vi "Design N IIR filters.vi"(4 "arrOptionalFilterSpecs":T3(array[cluster]) {"PB Gain" format="%0.2f"; "SB Gain" format="%0.2f"; "Lower SB" format="%0.2p"; "Upper SB" format="%0.2f"; "Lower PB" format="%0.2p"; "Upper PB" format="%0.2f"}, 6 "arrFilterSpecs":T2(array[cluster]) {"PB Ripple" format="%0.2f"; "Lower Fc" format="%0.2p"; "SB Attenuation" format="%0.2f"; "Upper Fc" format="%0.2p"}, 7 "redesign filters":bool[](array[boolean]), 8 "error in":errorcluster, 10 "filter structure option":T1=10 items=["IIR 2nd Order"=0, "IIR 4th Order"=1, "Auto Select"=10], 11 "arrdt":dbl[](array[numeric]) format="%0.2f") -> (0 "error out":errorcluster, 1 "arrIIRFilterCluster":T4(array[cluster]) {"Forward Coefficients" format="%0.2f"; "Reverse Coefficients" format="%0.2f"}, 3 "arrFilterInfo":T5(array[cluster]) {"phase H(w)"."df" format="%0.2f"; "phase H(w)"."f0" format="%0.2f"; "phase H(w)"."Phase H(w)" format="%0.2f"; "magnitude H(w)"."df" format="%0.2f"; "magnitude H(w)"."f0" format="%0.2f"; "magnitude H(w)"."Mag H(w)" format="%0.2f"}, 5 "reset filter states":bool[](array[boolean]))   [LabVIEW 2020, in "NI_MAPro.lvlib"]
uses:
  NI_MAPro.lvlib
  Filter Structure Type.ctl
  NI_MABase.lvlib
  NI_AALBase.lvlib
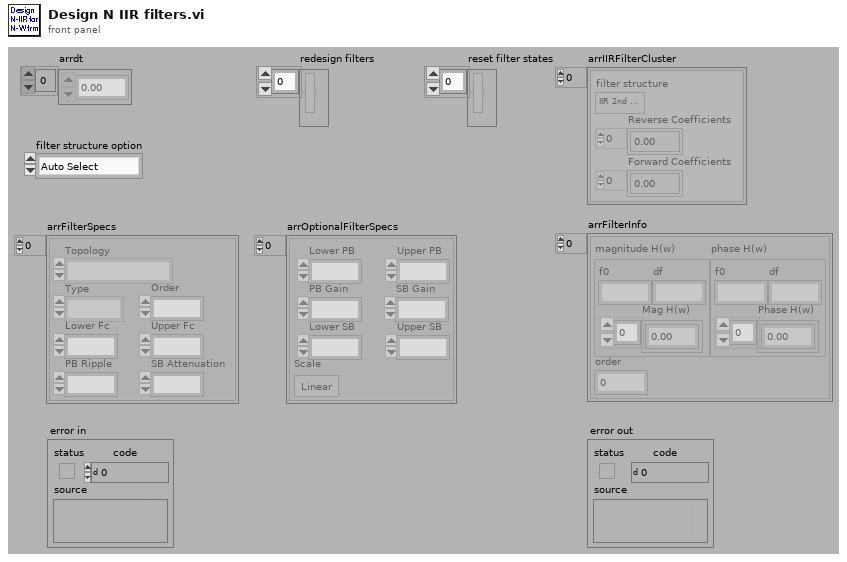
[diagram p1: front panel]
types:
  T1 = typedef "NI_AALBase.lvlib/Filter Structure Type.ctl" = u16
  T2 = cluster{"Topology":enum16{"Off", "Butterworth", "Chebyshev", "Inverse Chebyshev", "Elliptic", "Bessel"}, "Type":enum16{"Lowpass", "Highpass", "Bandpass", "Bandstop"}, "Order":i32, "Lower Fc":dbl, "Upper Fc":dbl, "PB Ripple":dbl, "SB Attenuation":dbl}[]
  T3 = cluster{"Lower PB":dbl, "Upper PB":dbl, "Lower SB":dbl, "Upper SB":dbl, "PB Gain":dbl, "SB Gain":dbl, "Scale":bool}[]
  T4 = cluster{"filter structure":enum32{"IIR 2nd Order", "IIR 4th Order"}, "Reverse Coefficients":dbl[], "Forward Coefficients":dbl[]}[]
  T5 = cluster{"magnitude H(w)":cluster{"f0":dbl, "df":dbl, "Mag H(w)":dbl[]}, "phase H(w)":cluster{"f0":dbl, "df":dbl, "Phase H(w)":dbl[]}, "order":i32}[]
  T6 = cluster{"Lower PB":dbl, "Upper PB":dbl, "Lower SB":dbl, "Upper SB":dbl, "PB Gain":dbl, "SB Gain":dbl, "Scale":bool}
  T7 = cluster{"magnitude H(w)":cluster{"f0":dbl, "df":dbl, "Mag H(w)":dbl[]}, "phase H(w)":cluster{"f0":dbl, "df":dbl, "Phase H(w)":dbl[]}, "order":i32}
  T8 = cluster{"filter structure":enum32{"IIR 2nd Order", "IIR 4th Order"}, "Reverse Coefficients":dbl[], "Forward Coefficients":dbl[]}
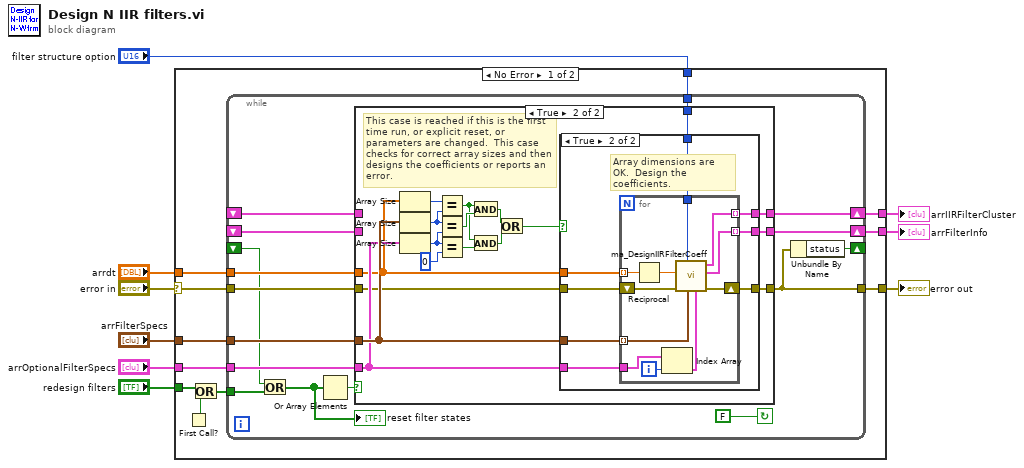
[diagram p0: block diagram]
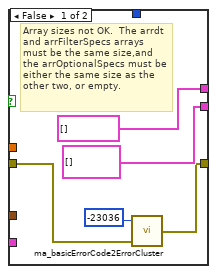
[diagram p3: hidden frame]
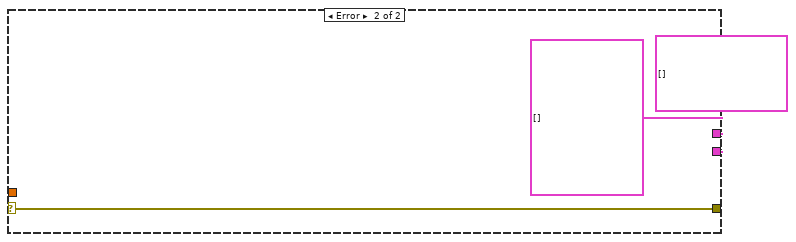
[diagram p4: hidden frame]
diagram:
  n1 = case shown="No Error" "error in" {
    selector: "error in" -> [w19 w84]
    tunnel: [w20 w84] -> w9
    tunnel: [w18 T5 []] -> w7
    tunnel: [w17 T4 []] -> w6
    tunnel: "arrOptionalFilterSpecs" -> [w16 _]
    tunnel: "arrFilterSpecs" -> [w15 _]
    tunnel: "arrdt" -> [w14 _]
    tunnel: "redesign filters" -> [w13 _]
    tunnel: "filter structure option" -> [w10 _]
    frame No Error {
      n2 = First Call?() -> (First Call?: T/F=w11:bool)
      n3 = Or(x=w13, y=w11) -> (x .or. y?=w12:bool[])
      n4 = while {
        tunnel: w14 -> [w31]
        tunnel: w15 -> [w30]
        tunnel: w16 -> [w29]
        tunnel: w19 -> [w27]
        tunnel: [w26] -> w20
        shift-left: _ -> [w33]
        shift-right: [w34] -> w18
        shift-left: _ -> [w36]
        shift-right: [w32] -> w17
        tunnel: w12 -> [w23]
        shift-right: [w25] -> _
        shift-left: _ -> [w24]
        tunnel: w10 -> [w21]
        stop <- FALSE continue-if-true
        n5 = Or(x=w24, y=w23) -> (x .or. y?=w22:bool[])
        "reset filter states" <- w22
        n6 = Or Array Elements(Boolean array=w22) -> (logical OR=w28:bool)
        n7 = case shown="True" w28 {
          tunnel: w36 -> [w39 _]
          tunnel: [w38 w57] -> w34
          tunnel: w33 -> [w38 _]
          tunnel: [w39 w56] -> w32
          tunnel: [w37 w55] -> w26
          tunnel: w31 -> [_ w41]
          tunnel: w30 -> [_ w45]
          tunnel: w29 -> [_ w44]
          tunnel: w27 -> [w37 w42]
          tunnel: w21 -> [_ w40]
          frame False {
            # "No change in parameters, no reset, and not the first time run."
          }
          frame True {
            # "This case is reached if this is the first time run, or explicit reset, or parameters are changed.  This case checks for correct array sizes and then designs the coefficients or reports an error."
            n8 = Array Size(array=w41) -> (size(s)=w54:i32)
            n9 = Array Size(array=w45) -> (size(s)=w53:i32)
            n10 = Array Size(array=w44) -> (size(s)=w51:i32)
            n11 = Equal?(x=w54, y=w53) -> (x = y?=w48:bool)
            n12 = Equal?(x=w53, y=w51) -> (x = y?=w52:bool)
            n13 = Equal?(x=w51, y=0) -> (x = y?=w49:bool)
            n14 = And(x=w48, y=w52) -> (x .and. y?=w47:bool)
            n15 = And(x=w48, y=w49) -> (x .and. y?=w46:bool)
            n16 = Or(x=w47, y=w46) -> (x .or. y?=w43:bool)
            n17 = case shown="True" w43 {
              tunnel: [T5 [] w70] -> w57
              tunnel: [T4 [] w69] -> w56
              tunnel: [w58 w68] -> w55
              tunnel: w41 -> [_ w67]
              tunnel: w45 -> [_ w66]
              tunnel: w44 -> [_ w65]
              tunnel: w42 -> [w60 w64]
              tunnel: w40 -> [_ w63]
              frame False {
                # "Array sizes not OK.  The arrdt and arrFilterSpecs arrays must be the same size,and the arrOptionalSpecs must be either the same size as the other two, or empty."
                n18 = call "ma_basicErrorCode2ErrorCluster.vi"("error in (no error)"=w60, "Error Code"=-23036) -> ("error out"=w58:errorcluster)  [unwired: 1 in]
              }
              frame True {
                # "Array dimensions are OK.  Design the coefficients."
                n19 = for {
                  tunnel: w66 -> [w72] mode=indexing
                  tunnel: [w81] -> w69 mode=indexing
                  tunnel: w65 -> [w79]
                  tunnel: w67 -> [w73] mode=indexing
                  tunnel: [w76] -> w70 mode=indexing
                  shift-right: [w75] -> w68
                  shift-left: w64 -> [w74]
                  tunnel: w63 -> [w71]
                  i -> [w77]
                  n20 = Reciprocal(x=w73) -> (1/x=w80:dbl)
                  n21 = Index Array(array=w79, index=w77) -> (element=w78:T6)
                  n22 = call "ma_DesignIIRFilterCoeff.vi"("Optional Filter Specifications"=w78, "Filter specifications"=w72, "filter structure option"=w71, "error in (no error)"=w74, "Sampling Frequency"=w80) -> ("error out"=w75:errorcluster, "Filter Information"=w76:T7, "IIR Filter Cluster"=w81:T8)  [unwired: 4 in]
                }
              }
            }
          }
        }
        n23 = Unbundle By Name(w26) -> ("status"=w25:bool)
      }
    }
    frame Error {
    }
  }
  "error out" <- w9
  "arrIIRFilterCluster" <- w6
  "arrFilterInfo" <- w7
